vi "Periodic Tasks.vi"(8 "error in":errorcluster) -> ()   [LabVIEW 2019]
doc: "This VI runs in parallel to other tasks. It can contain as many user-defined periodic loops as you need. These can carry out PID or other sorts of timed response."
panel:
  out "Connected?":bool
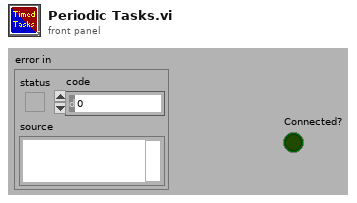
[diagram p1: front panel]
types:
  T1 = typedef "WPI_AnalogChannelDevRef.ctl" = cluster{"DevStatus":errorcluster, "Analog Channel":T2}
  T2 = typedef "FPGA_AIChannel.ctl" = enum8{"AI 0", "AI 1", "AI 2", "AI 3", "AI MXP 0", "AI MXP 1", "AI MXP 2", "AI MXP 3", "Invalid"}
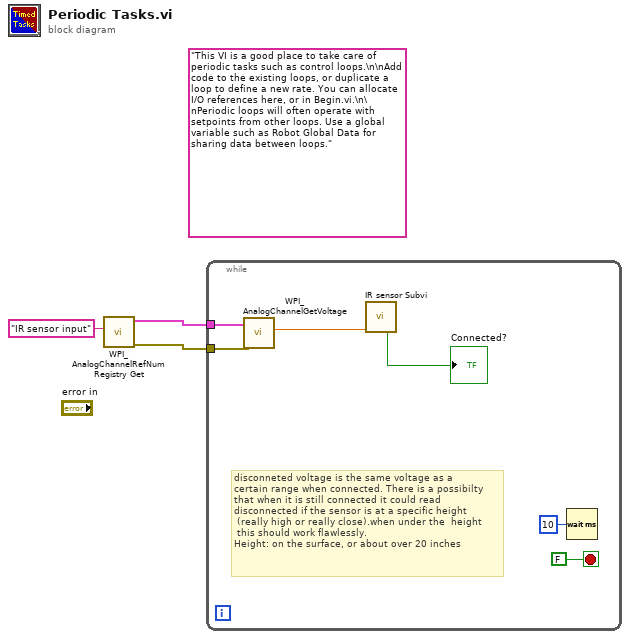
[diagram p0: block diagram]
diagram:
  (unwired) "This VI is a good place to take care of periodic tasks such as control loops.\n\nAdd code to the existing loops, or duplicate a loop to define a new rate. You can allocate I/O references here, or in Begin.vi.\n\nPeriodic loops will often operate with setpoints from other loops. Use a global variable such as Robot Global Data for sharing data between loops."
  n1 = call <vilib>:"WPI_AnalogChannelRefNum Registry Get.vi"("refnum name"="IR sensor input") -> ("error out"=w1:errorcluster, "AIDeviceRef"=w2:T1)  [unwired: 9 in]
  n2 = while {
    tunnel: w2 -> [w7]
    tunnel: w1 -> [w6]
    stop <- FALSE stop-if-true
    # "disconneted voltage is the same voltage as a\ncertain range when connected. There is a possibilty\nthat when it is still connected it could read \ndisconnected if the sensor is at a specific height\n (really high or really close).when under the  height\n this should work flawlessly.\nHeight: on the surface, or about over 20 inches"
    n3 = call <vilib>:"WPI_AnalogChannelGetVoltage.vi"("error in (no error)"=w6, "AIDeviceRef"=w7) -> ("Voltage"=w5:dbl)  [unwired: 7 in, 2 out]
    n4 = call "IR sensor Subvi.vi"("Numeric"=w5) -> ("Connected?"=→"Connected?":bool)  [unwired: 10 in]
    n5 = Wait (ms)(milliseconds to wait=u32 10) -> ()  [unwired: 1 out]
  }
